vi "proc_wait_exit.vi"(7 "timeout [ms]":i32, 8 "error in":errorcluster, 11 "process instance handle in":u32[](array[numeric])) -> (0 "error out":errorcluster, 2 "exit code":i32, 3 "process instance handle out":u32[](array[numeric]))   [LabVIEW 2012]
doc: "Waits for process instance exit code and closes handle afterwards. Be carefull using this without timeout (default) because it will hangup until process returnes. It DOES NOT terminates the process, it only waits until it finishes.\nCloses instance handles if proces exited."
panel:
  in  "code mem":i32
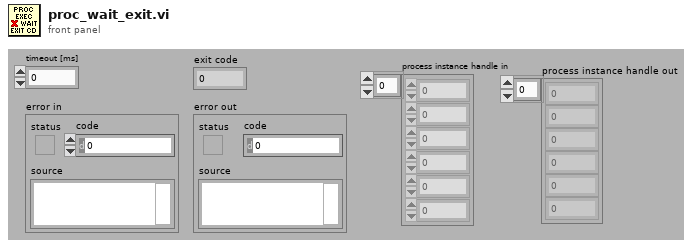
[diagram p1: front panel]
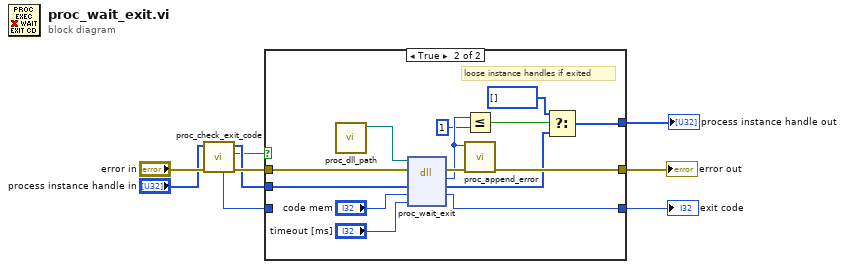
[diagram p0: block diagram]
diagram:
  n1 = call "proc_check_exit_code.vi"("error in"="error in", "instance handle in"="process instance handle in") -> ("error out"=w5:errorcluster, "running"=w2:bool, "instance handle out"=w4:u32[], "exit code"=w1:i32)  [unwired: 5 in, 1 out]
  n2 = case shown="True" w2 {
    tunnel: [w12 w26] -> w9
    tunnel: [w10 w21] -> w8
    tunnel: [w11 w18] -> w7
    tunnel: w5 -> [w12 w14]
    tunnel: w4 -> [w11 w13]
    tunnel: w1 -> [w10 _]
    frame False {
    }
    frame True {
      # "loose instance handles if exited"
      n3 = call "proc_dll_path.vi"() -> ("path out"=w25:path)  [unwired: 10 in, 1 out]
      n4 = dll-call lib="lv_proc.dll" fn="proc_wait_exit"(path in=w25, error in=w14, "proc"=w13, "code"="code mem", "timeout [ms]"="timeout [ms]") -> (error out=w24:errorcluster, "error"=w20:i32, "proc"=w16:u32[], "code"=w21:i32)  [unwired: 2 in, 1 out]
      n5 = Less Or Equal?(x=w20, y=1) -> (x <= y?=w17:bool)
      n6 = call "proc_append_error.vi"("error in"=w24, "code in"=w20) -> ("error out"=w26:errorcluster)  [unwired: 8 in, 1 out]
      n7 = Select(t=u32[] [], s=w17, f=w16) -> (s? t:f=w18:u32[])
    }
  }
  "error out" <- w9
  "process instance handle out" <- w7
  "exit code" <- w8
